vi "Basic FPGA IP module.vi"(4 "Input Valid":bool, 5 "Ready For Output":bool=TRUE, 6 "Range":cluster{"Lower Value":u8, "Upper Value":u8}={"Lower Value"=128, "Upper Value"=255}, 7 "Red Plane Out":T2) -> (3 "EdgeedPixels":T1)   [LabVIEW 2015]
doc: "Creates, edits, and runs vision algorithms using NI Vision Assistant.\n\nWhen you place this Express VI on the block diagram, NI Vision Assistant launches. Create an algorithm using the Vision Assistant processing functions. After you create an algorithm, you can select the controls and indicators that you want to be able to programmatically set in LabVIEW. Double-click the Vision Assistant Express VI to edit the algorithm."
uses:
  <vilib>/visionFPGA/Controls/IMAQ FPGA Pixel Bus u8x1.ctl
  <vilib>/visionFPGA/Controls/IMAQ FPGA Pixel Bus u1x1.ctl
  <vilib>/visionFPGA/NI_VDM_FPGA.lvlib
  <vilib>/visionFPGA/Process/Threshold/IMAQ FPGA Threshold U8 x1.vi
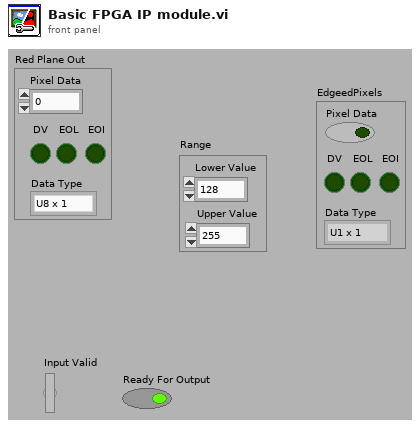
[diagram p1: front panel]
types:
  T1 = typedef "IMAQ FPGA Pixel Bus u1x1.ctl" = cluster{"Pixel Data":bool, "DV":bool, "EOL":bool, "EOI":bool, "Data Type":enum16{"U1 x 1"}}
  T2 = typedef "IMAQ FPGA Pixel Bus u8x1.ctl" = cluster{"Pixel Data":u8, "DV":bool, "EOL":bool, "EOI":bool, "Data Type":enum16{"U8 x 1"}}
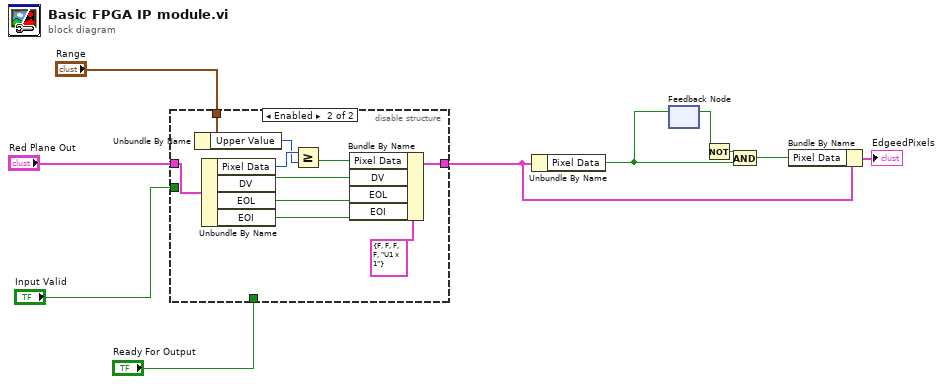
[diagram p0: block diagram]
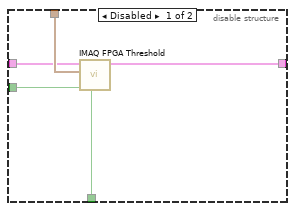
[diagram p2: hidden frame]
diagram:
  n1 = disable-structure shown="Enabled" {
    disable-tunnel: "Range" -> [w15 w25]
    disable-tunnel: "Ready For Output" -> [w14 _]
    disable-tunnel: "Red Plane Out" -> [w13 w24]
    disable-tunnel: "Input Valid" -> [w12 _]
    disable-tunnel: [w11 w16] -> w3
    frame Disabled {
      n2 = call-poly <vilib>:"IMAQ FPGA Threshold.vi"("Ready For Output"=w14, "Input Valid"=w12, "Range"=w15, "Pixel Bus In"=w13) -> ("Pixel Bus Out"=w11:T1)  [unwired: 5 in, 2 out]
    }
    frame Enabled {
      n3 = Unbundle By Name(w25) -> ("Upper Value"=w22:u8)
      n4 = Unbundle By Name(w24) -> ("Pixel Data"=w23:u8, "DV"=w19:bool, "EOL"=w18:bool, "EOI"=w17:bool)
      n5 = Greater Or Equal?(x=w23, y=w22) -> (x >= y?=w20:bool)
      n6 = Bundle By Name(cluster=T1 {"Pixel Data"=FALSE, "DV"=FALSE, "EOL"=FALSE, "EOI"=FALSE, "Data Type"=enum."U1 x 1"} ("Pixel Bus Out"), "Pixel Data"=w20, "DV"=w19, "EOL"=w18, "EOI"=w17) -> (w16:T1)
    }
  }
  n7 = Unbundle By Name(w3) -> ("Pixel Data"=w6:bool)
  n8 = feedback-in #1(w6) -> ()
  n9 = feedback #1() -> (w5:bool)  [unwired: 1 in]
  n10 = Not(x=w5) -> (.not. x?=w4:bool)
  n11 = And(x=w4, y=w6) -> (x .and. y?=w2:bool)
  n12 = Bundle By Name(cluster=w3, "Pixel Data"=w2) -> (→"EdgeedPixels":T1)
